vi "Read Array CAN.vi"(6 "timeout in ms (-1)":i32=-1, 8 "error in":errorcluster, 10 "COB IDs":u8[](array[numeric]) format="%x", 11 "CAN Session In":T2) -> (0 "error out":errorcluster, 2 "CAN Frame Out":T1 {"Data" format="%.0x"; "DataLength" format="%.0x"; "InfoB" format="%.0x"; "InfoA" format="%.0x"; "Type" format="%.0x"; "Identifier" format="%.0x"; "Timestamp" format="%.0x"}, 3 "CAN Session Out":T2)   [LabVIEW 2016]
doc: "The VI read a CAN packet (frame) from the CAN bus."
uses:
  Program Files (x86)/National Instruments/LabVIEW 2016/examples/robotics/EPOS2 CANOpen Driver/Low Level VIs/Typedefs/CAN Refnum.ctl
  Program Files (x86)/National Instruments/LabVIEW 2016/examples/robotics/EPOS2 CANOpen Driver/Low Level VIs/Typedefs/CAN Session Pointer.ctl
  Program Files (x86)/National Instruments/LabVIEW 2016/examples/robotics/EPOS2 CANOpen Driver/Low Level VIs/Typedefs/CAN Communication References.ctl
  Program Files (x86)/National Instruments/LabVIEW 2016/examples/robotics/EPOS2 CANOpen Driver/Low Level VIs/Typedefs/kill process notifier array.ctl
  Program Files (x86)/National Instruments/LabVIEW 2016/examples/robotics/EPOS2 CANOpen Driver/Low Level VIs/Typedefs/Write Queue.ctl
  Program Files (x86)/National Instruments/LabVIEW 2016/examples/robotics/EPOS2 CANOpen Driver/Low Level VIs/Typedefs/FPGA CAN Frame Cluster.ctl
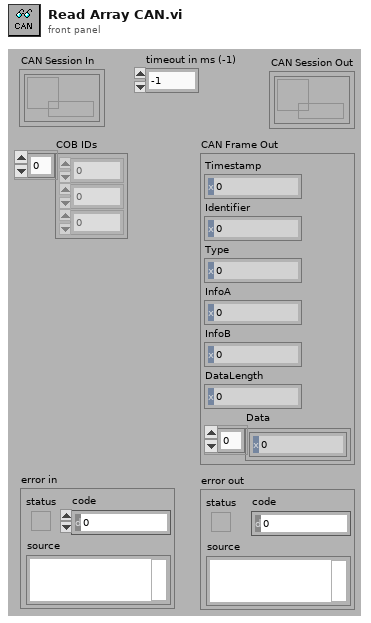
[diagram p1: front panel]
types:
  T1 = typedef "FPGA CAN Frame Cluster.ctl" = cluster{"Timestamp":u64, "Identifier":u32, "Type":u8, "InfoA":u8, "InfoB":u8, "DataLength":u8, "Data":u8[]}
  T2 = typedef "CAN Refnum.ctl" = refnum<k1>
  T3 = typedef "Write Queue.ctl" = refnum<queue>
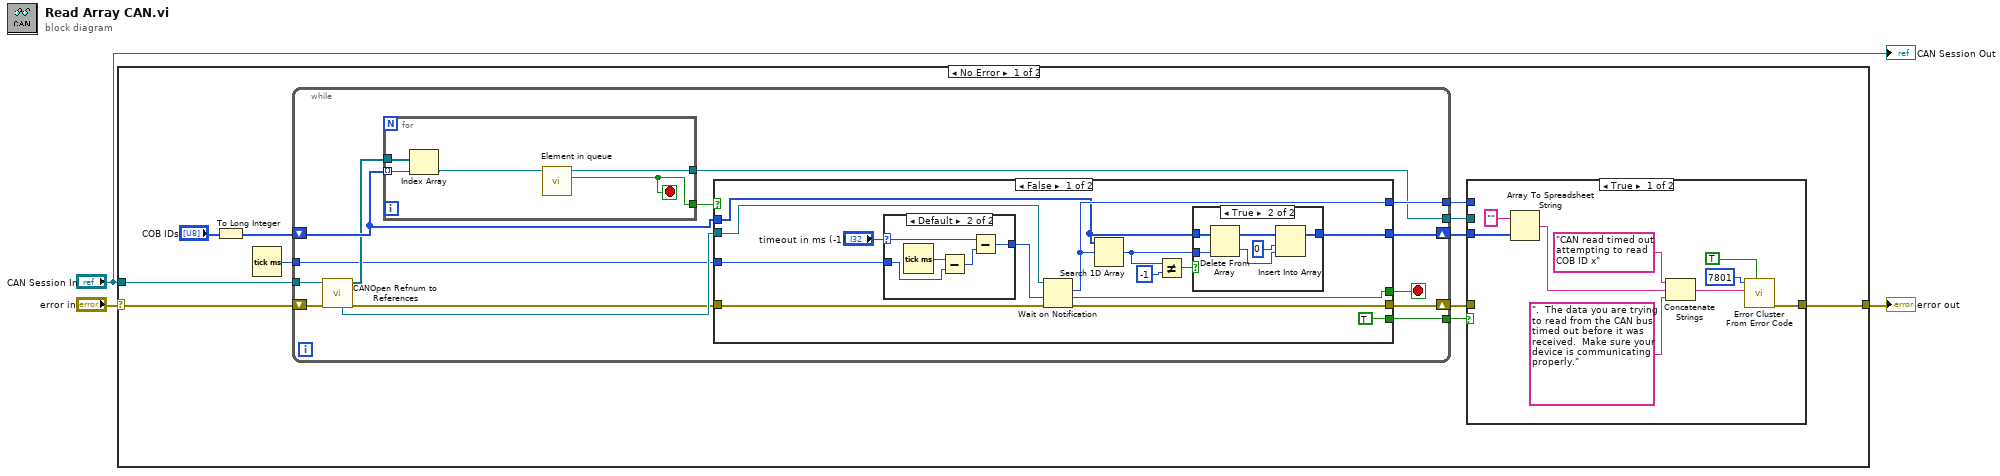
[diagram p0: block diagram]
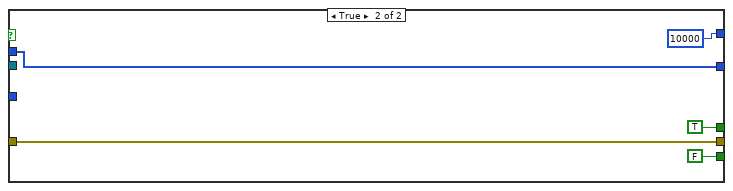
[diagram p4: hidden frame]
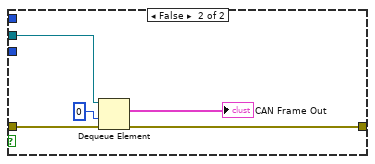
[diagram p5: hidden frame]
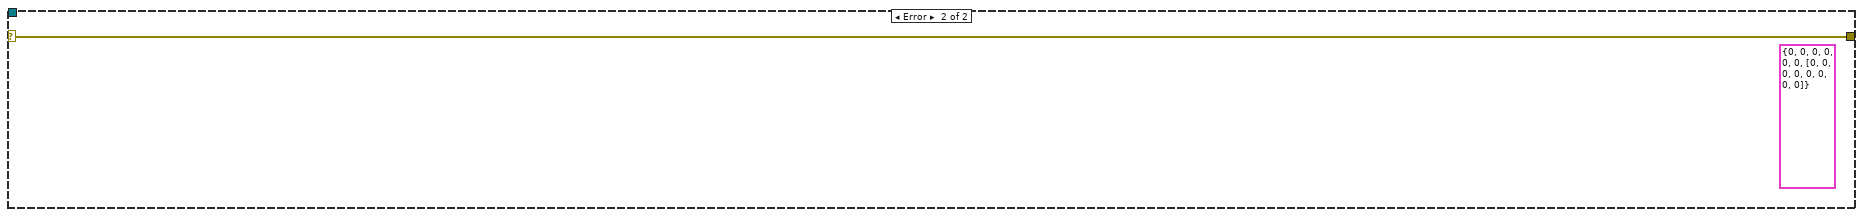
[diagram p6: hidden frame]
diagram:
  n1 = case shown="No Error" "error in" {
    selector: "error in" -> [w6 w80]
    tunnel: [w9 w80] -> w3
    tunnel: "CAN Session In" -> [w14 _]
    frame No Error {
      n2 = To Long Integer(number="COB IDs") -> (32bit integer=w13:i32[])
      n3 = Tick Count (ms)() -> (millisecond timer value=w5:u32)
      n4 = while {
        tunnel: w14 -> [w28]
        tunnel: [w26] -> w12
        tunnel: [w15] -> w10
        tunnel: [w23] -> w7
        shift-right: [w24] -> w8
        shift-left: w13 -> [w27]
        tunnel: w5 -> [w17]
        shift-right: [w25] -> w11
        shift-left: w6 -> [w19]
        stop <- w16 stop-if-true
        n5 = call "CANOpen Refnum to References.vi"("error in (no error)"=w19, "CAN Session In"=w28) -> ("error out"=w20:errorcluster, "Read Queue Array"=w21:T3[], "New Frame Notifier"=w22:refnum<notifier>)  [unwired: 7 out]
        n6 = for {
          tunnel: w27 -> [w65] mode=indexing
          tunnel: w21 -> [w64]
          tunnel: [w63] -> w18
          tunnel: [w62] -> w15
          stop <- w63 stop-if-true
          n7 = Index Array(array=w64, index=w65) -> (element=w61:T3)
          n8 = call "Element in queue.vi"("queue"=w61) -> ("Ready to read"=w63:bool, "queue out"=w62:T3)  [unwired: 9 in]
        }
        n9 = case shown="False" w18 {
          tunnel: [TRUE FALSE] -> w26
          tunnel: [w32 w60] -> w25
          tunnel: w22 -> [w42 _]
          tunnel: w27 -> [w37 w58]
          tunnel: w20 -> [w33 w60]
          tunnel: [w35 w58] -> w24
          tunnel: [w41 10000] -> w23
          tunnel: w17 -> [w34 _]
          tunnel: [w29 TRUE] -> w16
          frame False {
            n10 = case shown="Default" "timeout in ms (-1)" {
              selector: "timeout in ms (-1)" -> [w43 w44]
              tunnel: [w43 w48] -> w39
              tunnel: w34 -> [_ w46]
              frame -1 {
              }
              frame Default {
                n11 = Tick Count (ms)() -> (millisecond timer value=w47:u32)
                n12 = Subtract(x=w47, y=w46) -> (x-y=w45:u32)
                n13 = Subtract(x=w44, y=w45) -> (x-y=w48:u32)
              }
            }
            n14 = Wait on Notification(notifier=w42, timeout in ms (-1)=w39, error in (no error)=w33) -> (notification=w41:i32, timed out?=w29:bool, error out=w32:errorcluster)  [unwired: 1 in, 1 out]
            n15 = Search 1D Array(1D array=w37, element=w41) -> (index of element=w38:i32)  [unwired: 1 in]
            n16 = Not Equal?(x=w38, y=-1) -> (x != y?=w36:bool)
            n17 = case shown="True" w36 {
              tunnel: w38 -> [_ w54]
              tunnel: w37 -> [w49 w53]
              tunnel: [w49 w50] -> w35
              frame False {
              }
              frame True {
                n18 = Delete From Array(array=w53, index=w54) -> (deleted portion=w51:i32, array with subset deleted=w52:i32[])  [unwired: 1 in]
                n19 = Insert Into Array(array=w52, index=0, new element=w51) -> (w50:i32[])
              }
            }
          }
          frame True {
          }
        }
      }
      n20 = case shown="True" w12 {
        tunnel: [w70 w77] -> w9
        tunnel: w11 -> [_ w76]
        tunnel: w10 -> [_ w78]
        tunnel: w8 -> [w66 _]
        tunnel: w7 -> [_ _]
        frame True {
          n21 = Array To Spreadsheet String(array=w66, 3:"" ("format string")) -> (spreadsheet string=w68:string)  [unwired: 1 in]
          n22 = Concatenate Strings("CAN read timed out attempting to read COB ID x", w68, ".  The data you are trying to read from the CAN bus timed out before it was received.  Make sure your device is communicating properly.") -> (w72:string)
          n23 = call <vilib>:"Error Cluster From Error Code.vi"("show call chain? (False)"=TRUE, "error message (\"\")"=w72, "error code (0)"=7801) -> ("error out"=w70:errorcluster)  [unwired: 1 in, 5 out]
        }
        frame False {
          n24 = Dequeue Element(queue=w78, timeout in ms (-1)=0, error in (no error)=w76) -> (element=→"CAN Frame Out":T1, error out=w77:errorcluster)  [unwired: 2 out]
        }
      }
    }
    frame Error {
      (unwired) T1 {"Timestamp"=0, "Identifier"=0, "Type"=0, "InfoA"=0, "InfoB"=0, "DataLength"=0, "Data"=[0, 0, 0, 0, 0, 0, 0, 0]} ("CAN Frame")
    }
  }
  "error out" <- w3
  "CAN Session Out" <- "CAN Session In"
